vi "Pre Launch Init.vi"(11 "uService Template in":refnum<class "Father of all uServices.lvclass">) -> (0 "error out":errorcluster, 3 "uService Template out":refnum<class "Father of all uServices.lvclass">)   [LabVIEW 2026, in "TALOS.lvlib" / "Father of all uServices.lvlib" / "Father of all uServices.lvclass"]
doc: "(<B>Filename</B>: Actor Framework.lvlib:Actor.lvclass:Pre Launch Init.vi)\n\nDefines behavior that occurs after the Launch Nested Actor method is invoked but before the actor's Actor Core method begins running.\n\nBy default, this method does nothing. A descendant class may override it to define behavior."
uses:
  Father of all uServices.lvclass
  Ancestor/Ancestor/Ancestor.lvclass
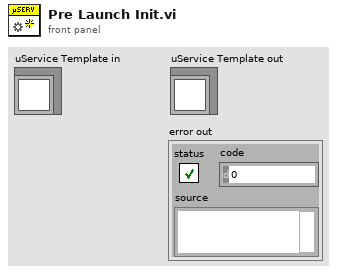
[diagram p1: front panel]
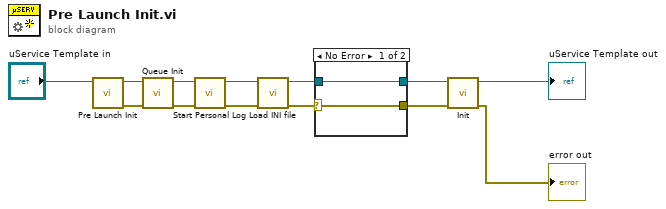
[diagram p0: block diagram]
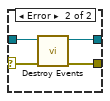
[diagram p2: hidden frame]
diagram:
  n1 = call-parent "Pre Launch Init.vi"("Ancestor in"="uService Template in") -> ("error out"=w11:errorcluster, "Ancestor out"=w10:refnum<class "Father of all uServices.lvclass">)  [unwired: 9 in]
  n2 = call "Queue Init.vi"("error in (no error)"=w11, "Father of all uServices in"=w10) -> ("error out"=w5:errorcluster, "Father of all uServices out"=w6:refnum<class "Father of all uServices.lvclass">)  [unwired: 8 in]
  n3 = call-dynamic "Start Personal Log.vi"("error in (no error)"=w5, "Father of all uServices in"=w6) -> ("error out"=w2:errorcluster, "Father of all uServices out"=w4:refnum<class "Father of all uServices.lvclass">)  [unwired: 8 in]
  n4 = call-dynamic "Load INI file.vi"("error in (no error)"=w2, "Father of all uServices in"=w4) -> ("error out"=w1:errorcluster, "Father of all uServices out"=w3:refnum<class "Father of all uServices.lvclass">)  [unwired: 8 in]
  n5 = case shown="No Error" w1 {
    selector: w1 -> [w15 w18]
    tunnel: [w14 w19] -> w8
    tunnel: [w15 w17] -> w7
    tunnel: w3 -> [w14 w16]
    frame No Error {
    }
    frame Error {
      n6 = call-dynamic "Destroy Events.vi"("error in (no error)"=w18, "uService Template in"=w16) -> ("error out"=w17:errorcluster, "uService Template out"=w19:refnum<class "Father of all uServices.lvclass">)  [unwired: 8 in]
    }
  }
  n7 = call-dynamic "Init.vi"("error in (no error)"=w7, "uService Template in"=w8) -> ("error out"=→"error out":errorcluster, "uService Template out"=→"uService Template out":refnum<class "Father of all uServices.lvclass">)  [unwired: 8 in]
